vi "Clear HWI.vi"(8 "error in (no error)":errorcluster, 11 "Aerotech_Soloist in":refnum<class "Aerotech_Soloist.lvclass">) -> (0 "error out":errorcluster, 3 "Aerotech_Soloist out":refnum<class "Aerotech_Soloist.lvclass">)   [LabVIEW 2013, in "Aerotech_Soloist.lvclass"]
uses:
  Aerotech_Soloist.lvclass
  ParsedSWILine.ctl
  Aerotech_Soloist.lvclass/Aerotech_Soloist.ctl
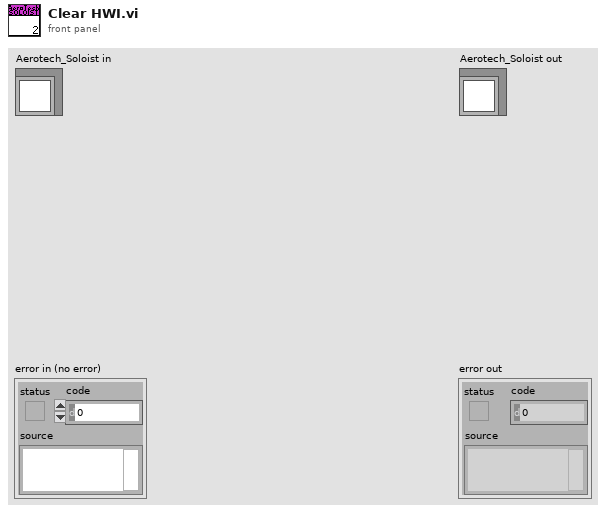
[diagram p1: front panel]
types:
  T1 = typedef "Aerotech_Soloist.lvclass/ParsedSWILine.ctl" = cluster{"ParameterScript":string, "CommandScript":string}
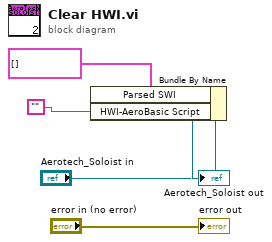
[diagram p0: block diagram]
diagram:
  n1 = Bundle By Name(cluster="Aerotech_Soloist in", "Parsed SWI"=T1[] [], "HWI-AeroBasic Script"="") -> (→"Aerotech_Soloist out":refnum<class "Aerotech_Soloist.lvclass">)
  "error out" <- "error in (no error)"
